vi "Get Compiled Counter And Protection Incoming Signals.vi"(0 "XNET Cluster":refnum<k21>, 5 "GUIDs":T13, 9 "Frames":T8 {"Frame Settings"."Transmit Trigger Ref" format="%.0x"; "Frame Settings"."Disable Transmission Ref" format="%.0x"; "Frame Refs" format="%.0x"}, 11 "error in (no error)":errorcluster) -> (3 "Incoming Signal Info":T2 {"Signal Settings Out"."Protection Configuration"."CRC Channels"."Data Type" items=["Signed", "Unsigned", "IEEE Float"]}, 4 "Incoming Frames":T12[](array[typedef]) {"Protection Configurations"."CRC Channels"."Data Type" items=["Signed", "Unsigned", "IEEE Float"]}, 6 "Incoming Signals Refs":T1[](array[typedef]) format="%.0x", 8 "Time Diff Refs":T1[](array[typedef]) format="%.0x", 10 "InvalidChannelRefs":T1[](array[typedef]) format="%.0x", 12 "All Signals Refs":T1[](array[typedef]) format="%.0x", 13 "Counters and Protection Refs":T1[](array[typedef]) format="%.0x", 14 "Receive Time Refs":T1[](array[typedef]) format="%.0x", 15 "error out":errorcluster)   [LabVIEW 2019]
uses:
  Types/Export Frame GUIDs List.ctl
  Shared/Types/Exported Frame Settings.ctl
  Shared/Types/Exported Frame Type.ctl
  Shared/Types/Exported Protection Settings.ctl
  Shared/Types/Protection Type.ctl
  Shared/Types/XNET Signal Configuration.ctl
  Shared/Types/Exported Counter Settings.ctl
  Shared/Types/Exported Event Trigger Type.ctl
  <vilib>/NI VeriStand/Custom Device API/Custom Device Item Ref.ctl
  Types/Export Frames List and Type.ctl
  Types/Exported Frame Settings.ctl
  Shared/Types/Incoming Signal Info.ctl
  Shared/Types/Exported Signal Settings.ctl
  Addon/Addon Shared/SubVIs/GUID Lookup.vi
  <vilib>/NI VeriStand/Custom Device Tools/Custom Device Utility Library/NI VeriStand - Search for All Items by GUID.vi
  <vilib>/NI VeriStand/Custom Device Tools/Custom Device Utility Library/NI VeriStand - Search for Item by GUID.vi
  Shared/Protection and Counter Support Shared.lvlib
  <vilib>/NI VeriStand/Custom Device API/Custom Device API.lvlib
  Protection and Counter Support System Explorer.lvlib
  <resource>/objmgr/xnet.rc
  <vilib>/NI VeriStand/Custom Device Tools/Custom Device Utility Library/Custom Device Utility Library.lvlib
  Addon/Addon Shared/Protection and Counter Addon Shared.lvlib
panel:
  in  "close VI":bool
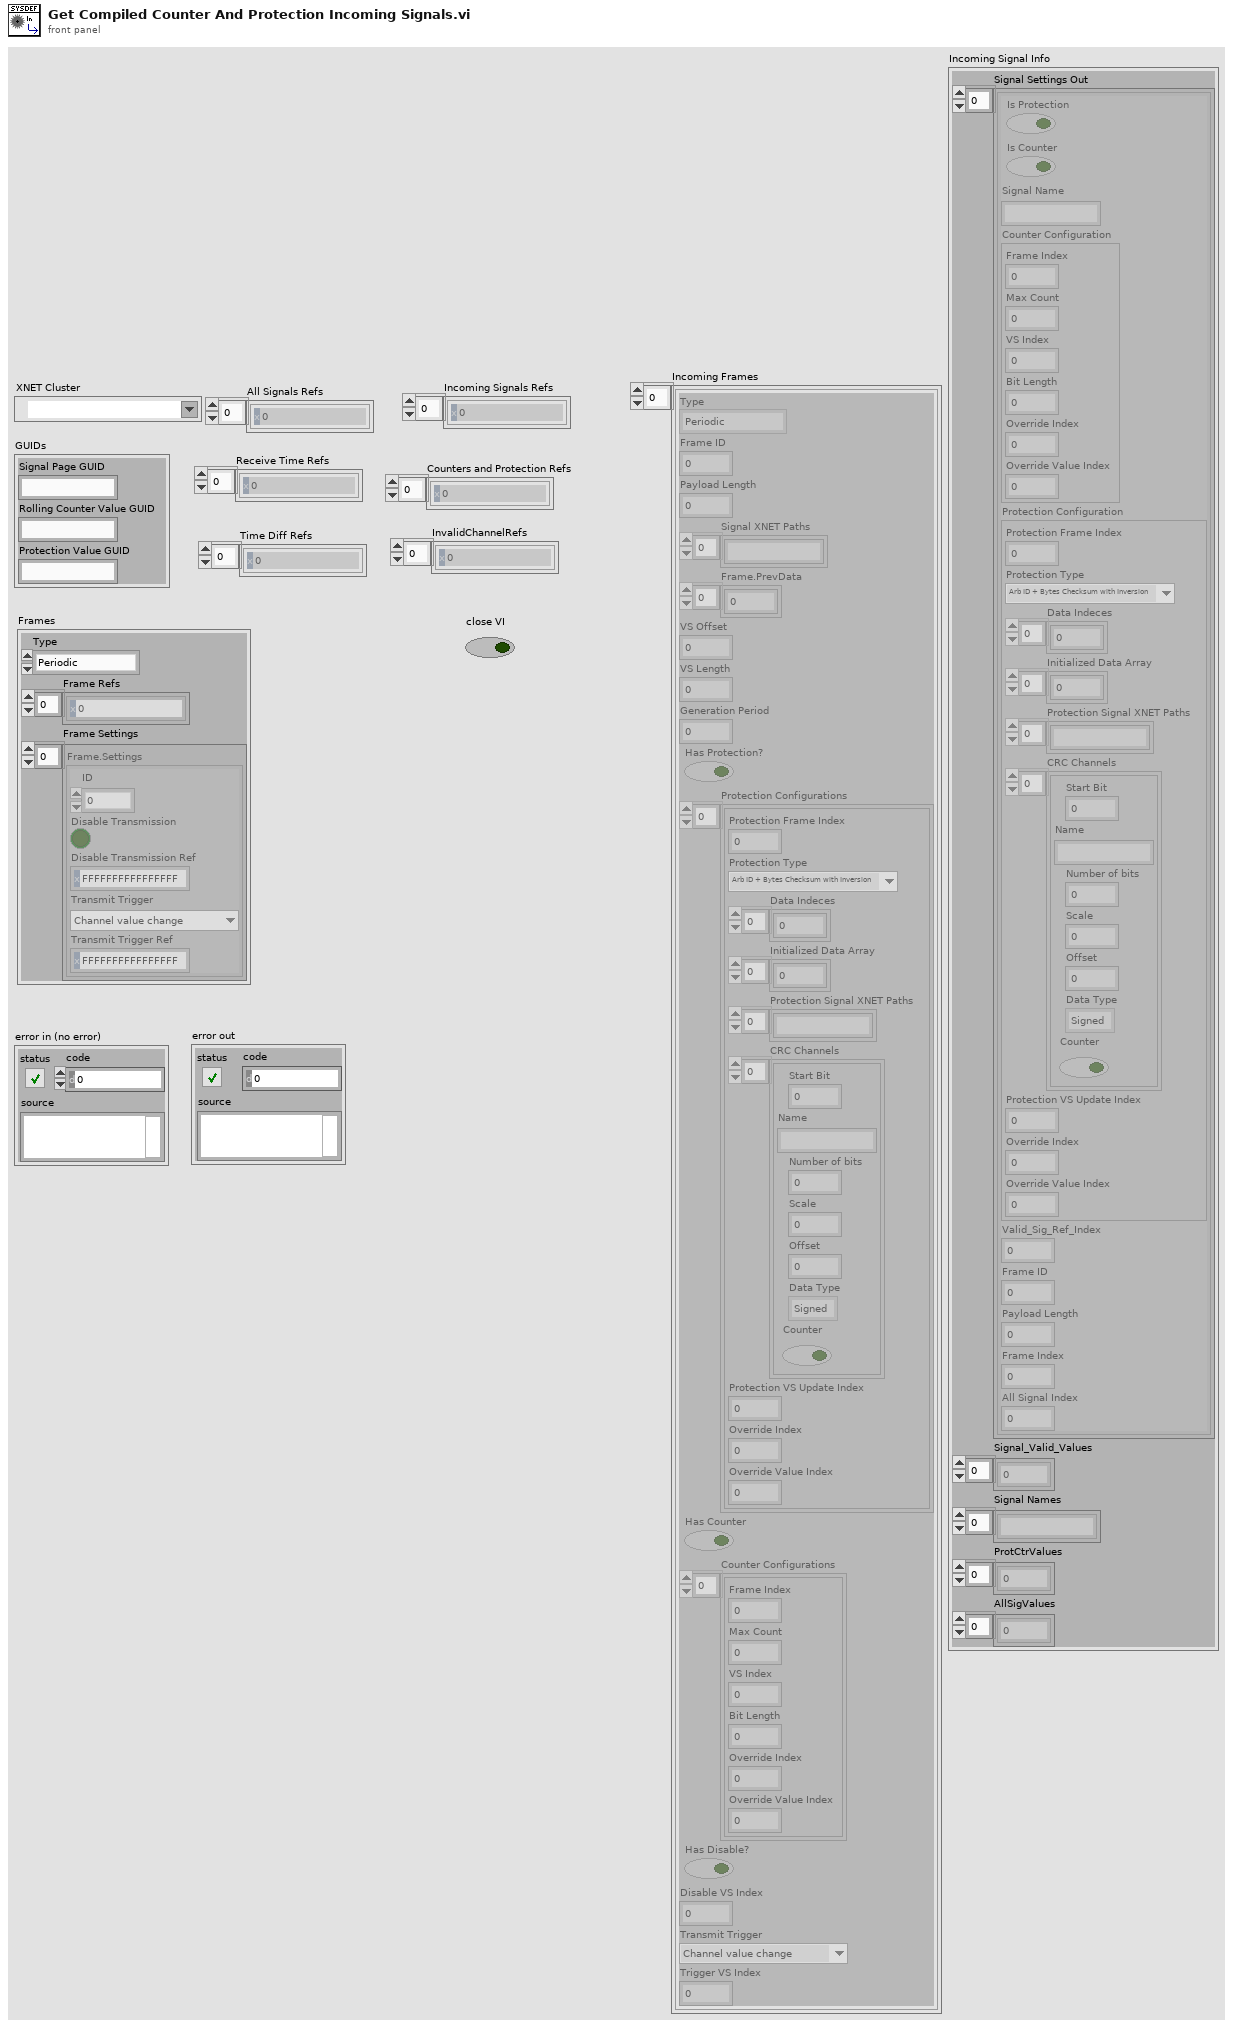
[diagram p1: front panel]
types:
  T1 = typedef "Custom Device API.lvlib/Custom Device Item Ref.ctl" = u64
  T2 = typedef "Incoming Signal Info.ctl" = cluster{"Signal Settings Out":T3[], "Signal_Valid_Values":dbl[], "Signal Names":string[], "ProtCtrValues":dbl[], "AllSigValues":dbl[]}
  T3 = typedef "Exported Signal Settings.ctl" = cluster{"Is Protection":bool, "Is Counter":bool, "Signal Name":string, "Counter Configuration":T4, "Protection Configuration":T5, "Valid_Sig_Ref_Index":i32, "Frame ID":u32, "Payload Length":u32, "Frame Index":i32, "All Signal Index":i32}
  T4 = typedef "Protection and Counter Support Shared.lvlib/Exported Counter Settings.ctl" = cluster{"Frame Index":i32, "Max Count":dbl, "VS Index":i32, "Bit Length":i64, "Override Index":i32, "Override Value Index":i32}
  T5 = typedef "Protection and Counter Support Shared.lvlib/Exported Protection Settings.ctl" = cluster{"Protection Frame Index":i32, "Protection Type":T6, "Data Indeces":i32[], "Initialized Data Array":dbl[], "Protection Signal XNET Paths":string[], "CRC Channels":T7[], "Protection VS Update Index":i32, "Override Index":i32, "Override Value Index":i32}
  T6 = typedef "Protection and Counter Support Shared.lvlib/Protection Type.ctl" = enum16{"Arb ID + Bytes Checksum with Inversion", "Arb ID + Bytes CRC with Inversion", "Reversed Raw Signal Checksum with Inversion", "Concatenated Two's Compliment"}
  T7 = typedef "Protection and Counter Support Shared.lvlib/XNET Signal Configuration.ctl" = cluster{"Start Bit":i32, "Name":string, "Number of bits":i32, "Scale":dbl, "Offset":dbl, "Data Type":u32, "Counter":bool}
  T8 = typedef "Protection and Counter Support System Explorer.lvlib/Export Frames List and Type.ctl" = cluster{"Type":T9, "Frame Refs":T1[], "Frame Settings":T10[]}
  T9 = typedef "Protection and Counter Support Shared.lvlib/Exported Frame Type.ctl" = enum16{"Periodic", "Event", "Periodic/Event"}
  T10 = typedef "Protection and Counter Support System Explorer.lvlib/Exported Frame Settings.ctl" = cluster{"ID":u32, "Disable Transmission":bool, "Disable Transmission Ref":T1, "Transmit Trigger":T11, "Transmit Trigger Ref":T1}
  T11 = typedef "Protection and Counter Support Shared.lvlib/Exported Event Trigger Type.ctl" = enum16{"Channel value change", "Trigger channel (not zero)", "Channel value change or trigger channel (not zero)", "Trigger channel (any value change)", "Channel value change or trigger channel (any value change)"}
  T12 = typedef "Protection and Counter Support Shared.lvlib/Exported Frame Settings.ctl" = cluster{"Type":T9, "Frame ID":u32, "Payload Length":u32, "Signal XNET Paths":string[], "Frame.PrevData":dbl[], "VS Offset":i32, "VS Length":i32, "Generation Period":u32, "Has Protection?":bool, "Protection Configurations":T5[], "Has Counter":bool, "Counter Configurations":T4[], "Has Disable?":bool, "Disable VS Index":i32, "Transmit Trigger":T11, "Trigger VS Index":i32}
  T13 = typedef "Protection and Counter Support System Explorer.lvlib/Export Frame GUIDs List.ctl" = cluster{"Signal Page GUID":string, "Rolling Counter Value GUID":string, "Protection Value GUID":string}
  T14 = typedef "Custom Device API.lvlib/Custom Device Item Info.ctl" = cluster{"Name":string, "Is Channel":bool, "GUID":string, "Is Waveform":bool}
  T15 = typedef "Protection and Counter Support System Explorer.lvlib/Protection Signal Settings.ctl" = cluster{"Input Channels":T16[], "Protection Type":T6}
  T16 = typedef "Protection and Counter Support System Explorer.lvlib/Protection Signal Linked Channel.ctl" = cluster{"Node Ref":T1}
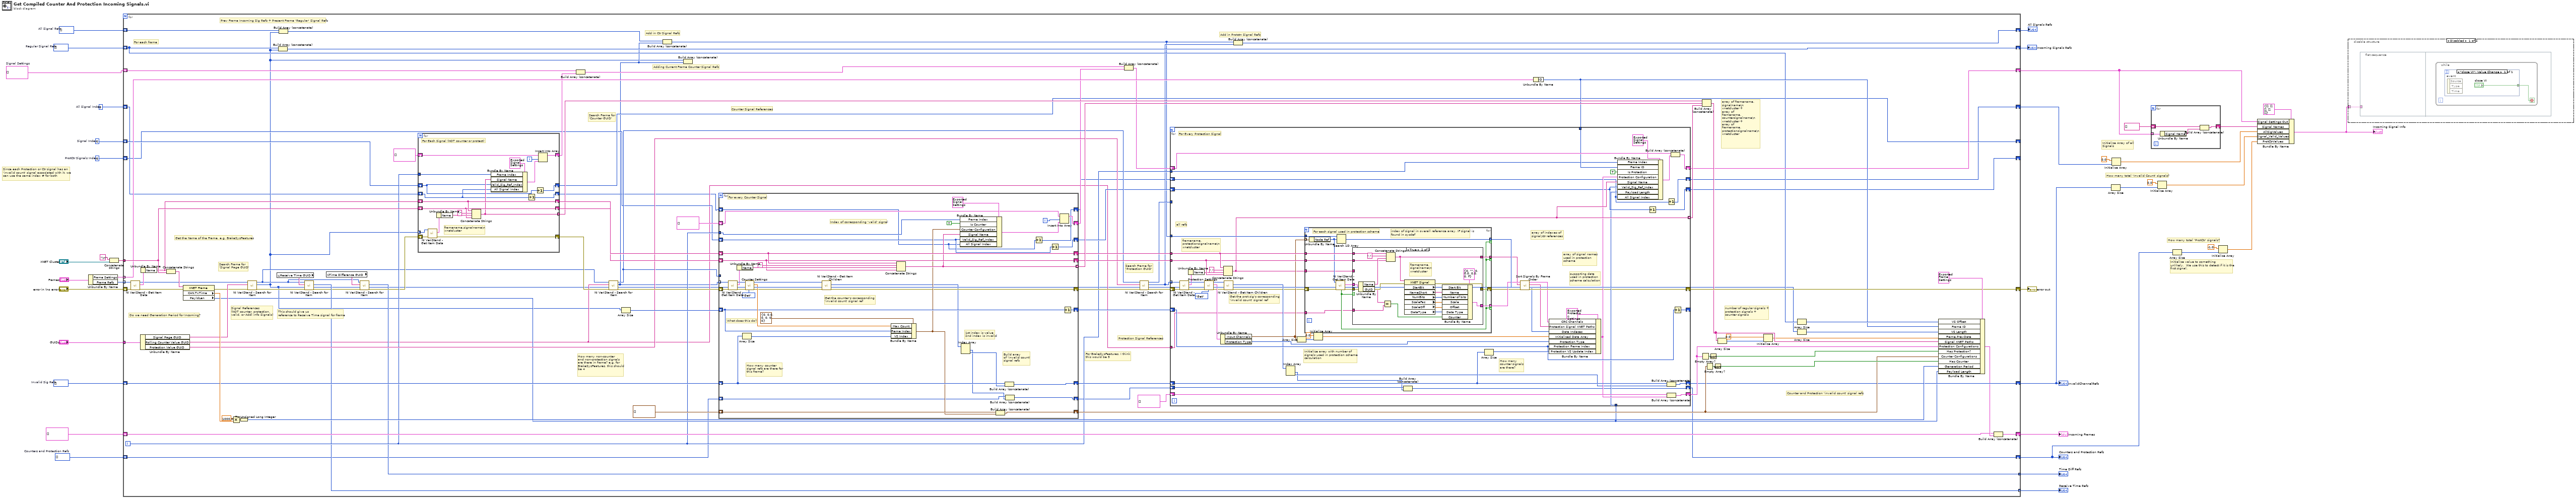
[diagram p0: block diagram]
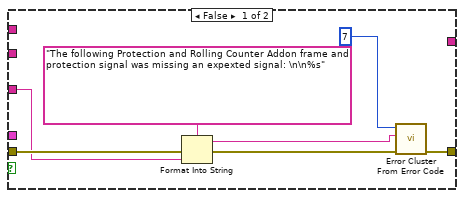
[diagram p3: hidden frame]
diagram:
  w6 = 0  # All Signal Index
  w8 = T1[] []  # All Signal Refs
  w12 = 0  # ProtCtr Signals Index
  w13 = 0  # Signal Index
  w17 = T1[] []  # Counters and Protection Refs
  w26 = T3[] []  # Signal Settings
  w37 = T1[] []  # Invalid Sig Refs
  w36 = T1[] []  # Regular Signal Refs
  # "Initialize value to something\nunlikely.  We use this to detect if it is the\nfirst signal."
  # "Initialize Array of all\nSignals"
  # "Since each Protection or Ctr signal has an\n'invalid count' signal associated with it, we \ncan use the same index # for both"
  # "How many total 'ProtCtr' signals?"
  # "How many total 'Invalid Count' signals?"
  n1 = Unbundle By Name("Frames") -> ("Frame Settings"=w29:T10[], "Frame Refs"=w30:T1[])
  n2 = Concatenate Strings("\n", "XNET Cluster") -> (w31:string)
  n3 = for {
    tunnel: w30 -> [w125] mode=indexing
    shift-right: [w98] -> w10
    shift-left: "error in (no error)" -> [w126]
    shift-right: [w51] -> w34
    shift-left: w36 -> [w69]
    tunnel: w31 -> [w112]
    shift-right: [w92] -> w9
    shift-left: w37 -> [w116]
    shift-right: [w90] -> w27
    shift-left: T12[] [] -> [w89]
    tunnel: "GUIDs" -> [w88]
    tunnel: w29 -> [w85] mode=indexing
    shift-right: [w70] -> w3
    shift-left: w26 -> [w81]
    tunnel: [w65] -> w20 mode=indexing
    tunnel: [w60] -> w18 mode=indexing
    shift-right: [w57] -> w11
    shift-left: w17 -> [w59]
    shift-right: [w55] -> _
    shift-left: w13 -> [w56]
    shift-right: [w53] -> _
    shift-left: w12 -> [w54]
    shift-right: [w45] -> w7
    shift-left: w8 -> [w48]
    shift-right: [w41] -> w4
    shift-left: w6 -> [w44]
    i -> [w68]
    # "Add in Protctn Signal Refs"
    # "Add in Ctr Signal Refs"
    # "This should give us\nreference to Receive Time signal for frame"
    # "Adding Current Frame Counter Signal Refs"
    # "Prev Frame Incoming Sig Refs + Present Frame 'Regular' Signal Refs"
    # "number of regular signals +\nprotection signals +\ncounter signals"
    # "array of framename.\nsignalname\\n\nxnetcluster + \narray of \nframename.\ncountersignalname\\n\nxnetcluster + \narray of \nframename.\nprotectionsignalname\\n\nxnetcluster"
    # "Counter and Protection 'invalid count' signal refs"
    # "For BrakeSysFeatures, I think \nthis would be 5"
    # "Protection Signal References"
    # "Search Frame for\n'Protection GUID'"
    # "Counter Signal References"
    # "Search Frame for\n'Counter GUID'"
    # "How many non-counter\nand non-protection signals\nare there in frame? e.g. for\nBrakeSysFeatures, this should\nbe 4"
    # "Signal References\n(NOT counter, protection, \nvalid, or Addl info Signals)"
    # "Search Frame for\n'Signal Page GUID'"
    # "Do we need Generation Period for Incoming?"
    # "Get the Name of the Frame, e.g. BrakeSysFeatures"
    # "For each frame"
    n4 = call <vilib>:"NI VeriStand - Get Item Data.vi"("error in (no error)"=w126, "Item Ref in"=w125) -> ("error out"=w122:errorcluster, "Item Info"=w124:T14, "Item Ref out"=w83:T1)  [unwired: 6 in, 1 out]
    n5 = Unbundle By Name(w88) -> ("Signal Page GUID"=w87:string, "Rolling Counter Value GUID"=w52:string, "Protection Value GUID"=w86:string)
    n6 = Unbundle By Name(w124) -> ("Name"=w111:string)
    n7 = Concatenate Strings(w111, w112) -> (w123:string)
    n8 = property class="XNET Frame"(reference=w123, error in=w122) -> (error out=w84:errorcluster, "CAN.TxTime"=w120:dbl, "PayldLen"=w71:u32)  [unwired: 1 out]
    n9 = Multiply(x=1000.0 ("y"), y=w120) -> (x*y=w121:dbl)
    n10 = To Unsigned Long Integer(number=w121) -> (unsigned 32bit integer=w118:u32)
    n11 = call-poly <vilib>:"NI VeriStand - Search for Item.vi"("error in"=w84, "Item GUID"=w87, "Section Ref in"=w83) -> ("error out"=w67:errorcluster, "Item Refs"=w47:T1[], "Section Ref out"=w61:T1)  [unwired: 5 in, 1 out]
    n12 = global read "GUID Lookup.vi" "Receive Time GUID"() -> (w66:string)
    n13 = Build Array (concatenate)(w69, w47) -> (w51:T1[])
    n14 = Build Array (concatenate)(w48, w47) -> (w46:T1[])
    n15 = call-poly <vilib>:"NI VeriStand - Search for Item.vi"("error in"=w67, "Item GUID"=w66, "Section Ref in"=w61) -> ("error out"=w64:errorcluster, "Item Ref"=w65:T1)  [unwired: 5 in, 2 out]
    n16 = global read "GUID Lookup.vi" "Time Difference GUID"() -> (w62:string)
    n17 = call-poly <vilib>:"NI VeriStand - Search for Item.vi"("error in"=w64, "Item GUID"=w62, "Section Ref in"=w61) -> ("error out"=w63:errorcluster, "Item Ref"=w60:T1)  [unwired: 5 in, 2 out]
    n18 = for {
      tunnel: w47 -> [w250] mode=indexing
      shift-right: [w245] -> w113
      shift-left: w63 -> [w249]
      tunnel: [w241] -> w108 mode=indexing
      shift-right: [w244] -> w110
      shift-left: w111 -> [w244]
      shift-right: [w243] -> w109
      shift-left: w112 -> [w243]
      shift-right: [w237] -> w80
      shift-left: T3[] [] -> [w240]
      tunnel: w68 -> [w236]
      shift-right: [w234] -> w55
      shift-left: w56 -> [w235]
      shift-right: [w233] -> w43
      shift-left: w44 -> [w232]
      i -> [w239]
      # "framename.signalname\\n\nxnetcluster"
      # "For Each Signal (NOT counter or protect)"
      n19 = call <vilib>:"NI VeriStand - Get Item Data.vi"("error in (no error)"=w249, "Item Ref in"=w250) -> ("error out"=w245:errorcluster, "Item Info"=w246:T14)  [unwired: 6 in, 2 out]
      n20 = Unbundle By Name(w246) -> ("Name"=w247:string)
      n21 = Concatenate Strings(w244, "." ("string"), w247, w243) -> (w241:string)
      n22 = Bundle By Name(cluster=T3 {"Is Protection"=FALSE, "Is Counter"=FALSE, "Signal Name"="", "Counter Configuration"={"Frame Index"=0, "Max Count"=0.0, "VS Index"=0, "Bit Length"=0, "Override Index"=0, "Override Value Index"=0}, "Protection Configuration"={"Protection Frame Index"=0, "Protection Type"=enum."Arb ID + Bytes Checksum with Inversion", "Data Indeces"=[], "Initialized Data Array"=[], "Protection Signal XNET Paths"=[], "CRC Channels"=[], "Protection VS Update Index"=0, "Override Index"=0, "Override Value Index"=0}, "Valid_Sig_Ref_Index"=0, "Frame ID"=0, "Payload Length"=0, "Frame Index"=0, "All Signal Index"=0} ("Signal Settings"), "Frame Index"=w236, "Signal Name"=w241, "Valid_Sig_Ref_Index"=w235, "All Signal Index"=w232) -> (w238:T3)
      n23 = Increment(x=w232) -> (x+1=w233:i32)
      n24 = Increment(x=w235) -> (x+1=w234:i32)
      n25 = Insert Into Array(array=w240, index=w239, new element=w238) -> (w237:T3[])
    }
    n26 = Build Array (concatenate)(w81, w80) -> (w77:T3[])
    n27 = call-poly <vilib>:"NI VeriStand - Search for Item.vi"("error in"=w113, "Item GUID"=w52, "Section Ref in"=w61) -> ("error out"=w115:errorcluster, "Item Refs"=w50:T1[], "Section Ref out"=w82:T1)  [unwired: 5 in, 1 out]
    n28 = Array Size(array=w47) -> (size(s)=w114:i32)
    n29 = Build Array (concatenate)(w46, w50) -> (w40:T1[])
    n30 = Build Array (concatenate)(w47, w50) -> ()  [unwired: 1 out]
    n31 = for {
      tunnel: w50 -> [w290] mode=indexing
      shift-right: [w258] -> w106
      shift-left: w115 -> [w289]
      shift-right: [w286] -> w127
      shift-left: T4[] [] -> [w285]
      tunnel: [w269] -> w107 mode=indexing
      shift-right: [w280] -> w93
      shift-left: w116 -> [w281]
      shift-right: [w275] -> w103
      shift-left: w114 -> [w276]
      shift-right: [w274] -> w101
      shift-left: w110 -> [w274]
      shift-right: [w273] -> w102
      shift-left: w109 -> [w273]
      tunnel: w82 -> [_]
      shift-right: [w264] -> w76
      shift-left: T3[] [] -> [w267]
      shift-right: [w263] -> w74
      shift-left: w54 -> [w262]
      tunnel: w68 -> [w261]
      shift-right: [w255] -> w58
      shift-left: w59 -> [w254]
      shift-right: [w251] -> w42
      shift-left: w43 -> [w252]
      i -> [w266]
      # "1st index is value\n2nd index is invalid"
      # "Index of corresponding 'valid' signal"
      # "Get the counter's corresponding\n'invalid count' signal ref"
      # "How many counter\nsignal refs are there for\nthis frame?"
      # "What does this do?"
      # "Build array\nof 'invalid count'\nsignal refs"
      # "For every Counter Signal"
      n32 = call <vilib>:"NI VeriStand - Get Item Data.vi"("error in (no error)"=w289, "Item Ref in"=w290) -> ("error out"=w287:errorcluster, "Item Info"=w282:T14, "Item Ref out"=w288:T1)  [unwired: 6 in, 1 out]
      n33 = Unbundle By Name(w282) -> ("Name"=w283:string)
      n34 = Array Size(array=w281) -> (size(s)=w277:i32)
      n35 = call "Counter Settings.vi"("Action"=enum8{"Get", "Set"}."Get", "error in"=w287, "Parent Ref"=w288) -> ("error out"=w259:errorcluster, "Max Count"=w279:dbl, "Parent Ref Out"=w260:T1)  [unwired: 6 in]
      n36 = call <vilib>:"NI VeriStand - Get Item Children.vi"("error in (no error)"=w259, "Item Ref in"=w260) -> ("error out"=w258:errorcluster, "Child Refs"=w257:T1[])  [unwired: 6 in, 2 out]
      n37 = Bundle By Name(cluster=T4 {"Frame Index"=0, "Max Count"=0.0, "VS Index"=0, "Bit Length"=0, "Override Index"=0, "Override Value Index"=0} ("Cluster"), "Max Count"=w279, "Frame Index"=w276, "VS Index"=w277) -> (w268:T4)
      n38 = Concatenate Strings(w274, "." ("string"), w283, w273) -> (w269:string)
      n39 = Bundle By Name(cluster=T3 {"Is Protection"=FALSE, "Is Counter"=FALSE, "Signal Name"="", "Counter Configuration"={"Frame Index"=0, "Max Count"=0.0, "VS Index"=0, "Bit Length"=0, "Override Index"=0, "Override Value Index"=0}, "Protection Configuration"={"Protection Frame Index"=0, "Protection Type"=enum."Arb ID + Bytes Checksum with Inversion", "Data Indeces"=[], "Initialized Data Array"=[], "Protection Signal XNET Paths"=[], "CRC Channels"=[], "Protection VS Update Index"=0, "Override Index"=0, "Override Value Index"=0}, "Valid_Sig_Ref_Index"=0, "Frame ID"=0, "Payload Length"=0, "Frame Index"=0, "All Signal Index"=0} ("Signal Settings"), "Frame Index"=w261, "Is Counter"=TRUE ("Is Protection"), "Counter Configuration"=w268, "Signal Name"=w269, "Valid_Sig_Ref_Index"=w262, "All Signal Index"=w252) -> (w265:T3)
      n40 = Index Array(array=w257) -> (element #1=w253:T1, element #2=w256:T1)  [unwired: 2 in]
      n41 = Build Array (concatenate)(w285, w268) -> (w286:T4[])
      n42 = Build Array (concatenate)(w281, w256) -> (w280:T1[])
      n43 = Build Array (concatenate)(w254, w253) -> (w255:T1[])
      n44 = Increment(x=w252) -> (x+1=w251:i32)
      n45 = Increment(x=w262) -> (x+1=w263:i32)
      n46 = Insert Into Array(array=w267, index=w266, new element=w265) -> (w264:T3[])
      n47 = Increment(x=w276) -> (x+1=w275:i32)
    }
    n48 = Build Array (concatenate)(w77, w76) -> (w75:T3[])
    n49 = call-poly <vilib>:"NI VeriStand - Search for Item.vi"("error in"=w106, "Item GUID"=w86, "Section Ref in"=w82) -> ("error out"=w105:errorcluster, "Item Refs"=w49:T1[], "Section Ref out"=w73:T1)  [unwired: 5 in, 1 out]
    n50 = Build Array (concatenate)(w40, w49) -> (w45:T1[])
    n51 = Unbundle By Name(w85) -> ("ID"=w72:u32)
    n52 = for {
      tunnel: w49 -> [w190] mode=indexing
      shift-right: [w140] -> w98
      shift-left: w105 -> [w189]
      shift-right: [w184] -> w99
      shift-left: T5[] [] -> [w186]
      tunnel: w40 -> [w185]
      tunnel: w101 -> [w182]
      tunnel: [w163] -> w100 mode=indexing
      shift-right: [w178] -> w92
      shift-left: w93 -> [w179]
      shift-right: [w168] -> _
      shift-left: w103 -> [w169]
      tunnel: w102 -> [w181]
      shift-right: [w159] -> w70
      shift-left: w75 -> [w165]
      shift-right: [w157] -> w53
      shift-left: w74 -> [w158]
      tunnel: w73 -> [_]
      tunnel: w72 -> [w156]
      tunnel: w71 -> [w155]
      tunnel: w68 -> [w154]
      shift-right: [w148] -> w57
      shift-left: w58 -> [w147]
      tunnel: w52 -> [w145]
      shift-right: [w135] -> w41
      shift-left: w42 -> [w136]
      # "Get the prot sig's corresponding\n'invalid count' signal ref"
      # "How many\ncounter signals\nare there?"
      # "Initialize array with number of \nsignals used in protection scheme\ncalculation"
      # "supporting data\nused in protection\nscheme calculation"
      # "array of signal names\nused in protection\nscheme"
      # "array of indexes of\nsignal/ctr references"
      # "all refs"
      # "For Every Protection Signal"
      # "framename.\nprotectionsignalname\\n\nxnetcluster"
      n53 = call <vilib>:"NI VeriStand - Get Item Data.vi"("error in (no error)"=w189, "Item Ref in"=w190) -> ("error out"=w187:errorcluster, "Item Info"=w180:T14, "Item Ref out"=w188:T1)  [unwired: 6 in, 1 out]
      n54 = Unbundle By Name(w180) -> ("Name"=w167:string)
      n55 = call "Protection Settings.vi"("Action"=enum8{"Get", "Set"}."Get", "error in"=w187, "Parent Ref"=w188) -> ("error out"=w151:errorcluster, "Selected Channels"=w177:T15, "Parent Ref Out"=w152:T1)  [unwired: 6 in]
      n56 = Unbundle By Name(w177) -> ("Input Channels"=w175:T16[], "Protection Type"=w176:T6)
      n57 = Concatenate Strings(w182, "." ("string"), w167, w181) -> (w163:string)
      n58 = call <vilib>:"NI VeriStand - Get Item Children.vi"("error in (no error)"=w151, "Item Ref in"=w152) -> ("error out"=w150:errorcluster, "Child Refs"=w153:T1[])  [unwired: 6 in, 2 out]
      n59 = Index Array(array=w153) -> (element #1=w146:T1, element #2=w149:T1)  [unwired: 2 in]
      n60 = Array Size(array=w175) -> (size(s)=w174:i32)
      n61 = for {
        tunnel: w185 -> [w195]
        tunnel: w175 -> [w205] mode=indexing
        tunnel: [w204] -> w144 mode=indexing if=w193
        shift-right: [w198] -> w141
        shift-left: w150 -> [w203]
        tunnel: w182 -> [w201]
        tunnel: w181 -> [w200]
        tunnel: [w196] -> w142 mode=indexing if=w193
        tunnel: [w197] -> w143 mode=indexing if=w193
        tunnel: w163 -> [w192]
        tunnel: w145 -> [w191]
        # "index of signal in overall reference array, IF signal is\nfound in sysdef"
        # "For each signal used in protection scheme"
        n62 = Unbundle By Name(w205) -> ("Node Ref"=w194:T1)
        n63 = call <vilib>:"NI VeriStand - Get Item Data.vi"("error in (no error)"=w203, "Item Ref in"=w194) -> ("error out"=w199:errorcluster, "Item Info"=w202:T14, "Found"=w193:bool)  [unwired: 6 in, 1 out]
        n64 = Search 1D Array(1D array=w195, element=w194) -> (index of element=w204:i32)  [unwired: 1 in]
        n65 = case shown="True" w193 {
          tunnel: w202 -> [_ w231]
          tunnel: w201 -> [_ w228]
          tunnel: w200 -> [_ w227]
          tunnel: w199 -> [w210 w226]
          tunnel: [w212 w225] -> w198
          tunnel: [_ w217] -> w197
          tunnel: [_ w216] -> w196
          tunnel: w192 -> [w207 _]
          tunnel: w191 -> [_ w214]
          frame False {
            n66 = Format Into String(format string="The following Protection and Rolling Counter Addon frame and protection signal was missing an expexted signal: \n\n%s" ("error message (\"\")"), error in=w210, w207) -> (resulting string=w206:string, error out=w209:errorcluster)  [unwired: 1 in]
            n67 = call <vilib>:"Error Cluster From Error Code.vi"("error in (no error)"=w209, "error message (\"\")"=w206, "error code (0)"=7) -> ("error out"=w212:errorcluster)  [unwired: 6 in]
          }
          frame True {
            # "framename.\nsignalname\\n\nxnetcluster"
            n68 = Unbundle By Name(w231) -> ("Name"=w229:string, "GUID"=w215:string)
            n69 = Equal?(x=w215, y=w214) -> (x = y?=w213:bool)
            n70 = Concatenate Strings(w228, "." ("string"), w229, w227) -> (w216:string)
            n71 = property class="XNET Signal"(reference=w216, error in=w226) -> (error out=w225:errorcluster, "StartBit"=w218:u32, "NameShort"=w219:string, "NumBits"=w220:u32, "ScaleFac"=w221:dbl, "ScaleOff"=w222:dbl, "DataType"=w223:u32)  [unwired: 1 out]
            n72 = Bundle By Name(cluster=T7 {"Start Bit"=0, "Name"="", "Number of bits"=0, "Scale"=0.0, "Offset"=0.0, "Data Type"=0, "Counter"=FALSE} ("MonitoredChannelSettings"), "Start Bit"=w218, "Name"=w219, "Number of bits"=w220, "Scale"=w221, "Offset"=w222, "Data Type"=w223, "Counter"=w213) -> (w217:T7)
          }
        }
      }
      n73 = Initialize Array(0.0 ("element"), w174) -> (w172:dbl[])
      n74 = Build Array (concatenate)(w147, w146) -> (w148:T1[])
      n75 = Array Size(array=w179) -> (size(s)=w170:i32)
      n76 = call "Sort Signals By Frame Order.vi"("error in (no error)"=w141, "Node Refs"=w144, "XNET Paths"=w142, "Signals"=w143) -> ("error out"=w140:errorcluster, "Ordered Node Refs"=w137:i32[], "Ordered XNET Paths"=w138:string[], "Ordered Signals"=w139:T7[])  [unwired: 4 in]
      n77 = Bundle By Name(cluster=T5 {"Protection Frame Index"=0, "Protection Type"=enum."Arb ID + Bytes Checksum with Inversion", "Data Indeces"=[], "Initialized Data Array"=[], "Protection Signal XNET Paths"=[], "CRC Channels"=[], "Protection VS Update Index"=0, "Override Index"=0, "Override Value Index"=0} ("Cluster"), "CRC Channels"=w139, "Protection Signal XNET Paths"=w138, "Data Indeces"=w137, "Initialized Data Array"=w172, "Protection Type"=w176, "Protection Frame Index"=w169, "Protection VS Update Index"=w170) -> (w161:T5)
      n78 = Bundle By Name(cluster=T3 {"Is Protection"=FALSE, "Is Counter"=FALSE, "Signal Name"="", "Counter Configuration"={"Frame Index"=0, "Max Count"=0.0, "VS Index"=0, "Bit Length"=0, "Override Index"=0, "Override Value Index"=0}, "Protection Configuration"={"Protection Frame Index"=0, "Protection Type"=enum."Arb ID + Bytes Checksum with Inversion", "Data Indeces"=[], "Initialized Data Array"=[], "Protection Signal XNET Paths"=[], "CRC Channels"=[], "Protection VS Update Index"=0, "Override Index"=0, "Override Value Index"=0}, "Valid_Sig_Ref_Index"=0, "Frame ID"=0, "Payload Length"=0, "Frame Index"=0, "All Signal Index"=0} ("Signal Settings"), "Frame Index"=w154, "Frame ID"=w156, "Is Protection"=TRUE, "Protection Configuration"=w161, "Signal Name"=w163, "Valid_Sig_Ref_Index"=w158, "Payload Length"=w155, "All Signal Index"=w136) -> (w160:T3)
      n79 = Increment(x=w158) -> (x+1=w157:i32)
      n80 = Build Array (concatenate)(w179, w149) -> (w178:T1[])
      n81 = Build Array (concatenate)(w186, w161) -> (w184:T5[])
      n82 = Increment(x=w136) -> (x+1=w135:i32)
      n83 = Build Array (concatenate)(w165, w160) -> (w159:T3[])
      n84 = Increment(x=w169) -> (x+1=w168:i32)
    }
    n85 = Empty Array?(array=w99) -> (empty?=w129:bool)
    n86 = Build Array (concatenate)(w108, w107, w100) -> (w97:string[])
    n87 = Empty Array?(array=w127) -> (empty?=w131:bool)
    n88 = Not(x=w129) -> (.not. x?=w128:bool)
    n89 = Not(x=w131) -> (.not. x?=w130:bool)
    n90 = Array Size(array=w97) -> (size(s)=w95:i32)
    n91 = Initialize Array(0.0 ("element"), w95) -> (w94:dbl[])
    n92 = Array Size(array=w69) -> (size(s)=w133:i32)
    n93 = Array Size(array=w47) -> (size(s)=w117:i32)
    n94 = Bundle By Name(cluster=T12 {"Type"=enum."Periodic", "Frame ID"=0, "Payload Length"=0, "Signal XNET Paths"=[], "Frame.PrevData"=[], "VS Offset"=0, "VS Length"=0, "Generation Period"=0, "Has Protection?"=FALSE, "Protection Configurations"=[], "Has Counter"=FALSE, "Counter Configurations"=[], "Has Disable?"=FALSE, "Disable VS Index"=0, "Transmit Trigger"=enum."Channel value change", "Trigger VS Index"=0} ("Frame Settings"), "VS Offset"=w133, "Frame ID"=w72, "VS Length"=w117, "Frame.PrevData"=w94, "Signal XNET Paths"=w97, "Protection Configurations"=w99, "Has Protection?"=w128, "Counter Configurations"=w127, "Has Counter"=w130, "Generation Period"=w118, "Payload Length"=w71) -> (w91:T12)
    n95 = Build Array (concatenate)(w89, w91) -> (w90:T12[])
  }
  "Incoming Frames" <- w27
  "error out" <- w10
  "InvalidChannelRefs" <- w9
  "Incoming Signals Refs" <- w34
  "Receive Time Refs" <- w20
  "Time Diff Refs" <- w18
  "Counters and Protection Refs" <- w11
  "All Signals Refs" <- w7
  n96 = Array Size(array=w9) -> (size(s)=w24:i32)
  n97 = Initialize Array(0.0 ("element"), w4) -> (w1:dbl[])
  n98 = for {
    tunnel: w3 -> [w294] mode=indexing
    shift-right: [w291] -> w2
    shift-left: string[] [] -> [w293]
    n99 = Unbundle By Name(w294) -> ("Signal Name"=w292:string)
    n100 = Build Array (concatenate)(w293, w292) -> (w291:string[])
  }
  n101 = Initialize Array(0.0 ("element"), w24) -> (w22:dbl[])
  n102 = Array Size(array=w11) -> (size(s)=w15:i32)
  n103 = Initialize Array(-1.0 ("element"), w15) -> (w14:dbl[])
  n104 = Bundle By Name(cluster=T2 {"Signal Settings Out"=[], "Signal_Valid_Values"=[], "Signal Names"=[], "ProtCtrValues"=[], "AllSigValues"=[]} ("Incoming Signal Info"), "Signal Settings Out"=w3, "Signal Names"=w2, "AllSigValues"=w1, "Signal_Valid_Values"=w22, "ProtCtrValues"=w14) -> (w19:T2)
  "Incoming Signal Info" <- w19
  n105 = disable-structure shown="Disabled" {
    disable-tunnel: w19 -> [w295 _]
    frame Disabled {
      n106 = flat-sequence {
        tunnel: w295 -> [_]
        frame #0 {
        }
        frame #1 {
          n107 = while {
            stop <- w296 stop-if-true
            n108 = event shown="[0] \"close VI\": Value Change" {
              selector: _ -> [_]
              dyn-events: _ -> [_]
              timeout: _ -> [_]
              tunnel: ["close VI"] -> w296
              event "close VI": Value Change {
                n109 = event-data() -> ()  [unwired: 1 in, 3 out]
              }
            }
          }
        }
      }
    }
    frame Enabled {
    }
  }
